vi "Geometry_Util_Test.vi"(8 "error in (no error)":errorcluster) -> (0 "error out":errorcluster, 3 "All Passed":bool)   [LabVIEW 2019]
uses:
  <vilib>/Rock Robotics/WPI/ThirdParty/JAS_Junk/TrajLib/Conv_Deg_Radians.vi
  <vilib>/Rock Robotics/WPI/ThirdParty/JAS_Junk/TrajLib/Rotation2d_CreateAngle.vi
  <vilib>/Rock Robotics/WPI/ThirdParty/JAS_Junk/TrajLib/Rotation2d_GetRadians.vi
  <vilib>/Rock Robotics/WPI/ThirdParty/JAS_Junk/TrajLib/Conv_Radians_Deg.vi
  <vilib>/Rock Robotics/WPI/ThirdParty/MJansen/PathPlanner/PathPlanner.lvlib
  <vilib>/Rock Robotics/WPI/ThirdParty/JAS_Junk/TrajLib/Trajectory_Library.lvlib
panel:
  out "Passed 5":bool
  out "Passed 4":bool
  out "Passed 3":bool
  out "Passed 2":bool
  out "Passed 1":bool
  # "Quadratic LERP"
  # "Double LERP"
  # "Rotational LERP"
  # "Cubic LERP"
  # "Translational LERP"
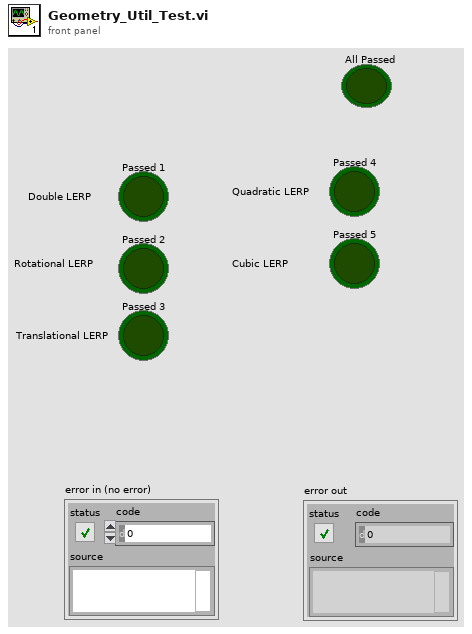
[diagram p1: front panel]
types:
  T1 = typedef "Trajectory_Library.lvlib/TRANSLATION2D.ctl" = cluster{"X":dbl, "Y":dbl}
  T2 = typedef "Trajectory_Library.lvlib/ROTATION2D.ctl" = cluster{"VALUE":dbl, "COS":dbl, "SIN":dbl}
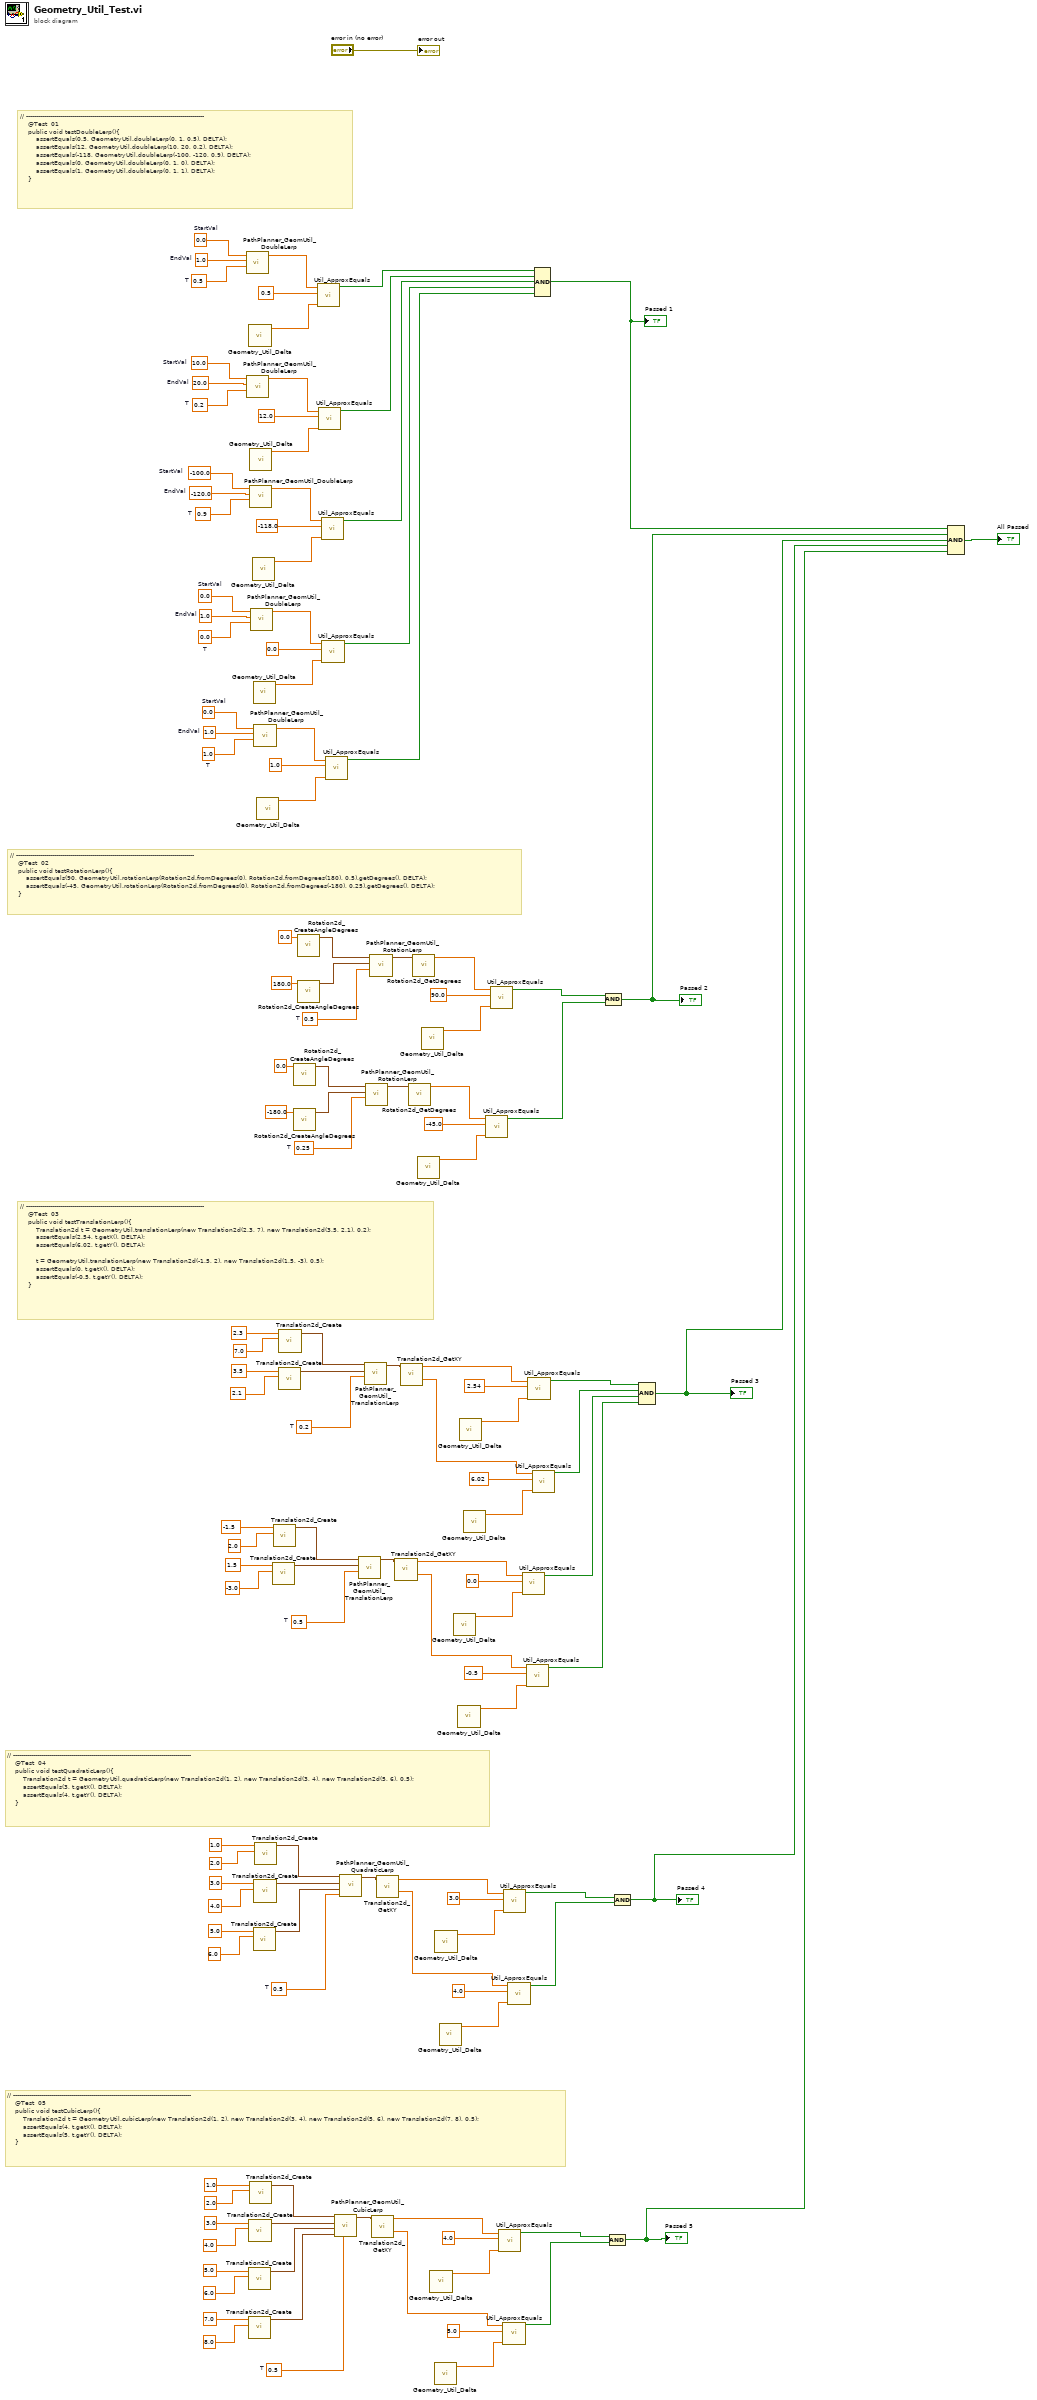
[diagram p0: block diagram]
diagram:
  w21 = 0.5  # T
  w41 = 0.5  # T
  w57 = 0.5  # T
  w74 = 0.2  # T
  w85 = 0.25  # T
  w95 = 0.5  # T
  w103 = 0.0  # StartVal
  w104 = 1.0  # EndVal
  w105 = 1.0  # T
  w109 = 0.0  # StartVal
  w110 = 1.0  # EndVal
  w111 = 0.0  # T
  w115 = -100.0  # StartVal
  w116 = -120.0  # EndVal
  w117 = 0.9  # T
  w121 = 10.0  # StartVal
  w122 = 20.0  # EndVal
  w123 = 0.2  # T
  w128 = 0.0  # StartVal
  w129 = 1.0  # EndVal
  w130 = 0.5  # T
  # "// -----------------------------------------------------------------------------------------\n    @Test  05\n    public void testCubicLerp(){\n        Translation2d t = GeometryUtil.cubicLerp(new Translation2d(1, 2), new Translation2d(3, 4), new Translation2d(5, 6), new Translation2d(7, 8), 0.5);\n        assertEquals(4, t.getX(), DELTA);\n        assertEquals(5, t.getY(), DELTA);\n    }"
  # "// -----------------------------------------------------------------------------------------\n    @Test  04\n    public void testQuadraticLerp(){\n        Translation2d t = GeometryUtil.quadraticLerp(new Translation2d(1, 2), new Translation2d(3, 4), new Translation2d(5, 6), 0.5);\n        assertEquals(3, t.getX(), DELTA);\n        assertEquals(4, t.getY(), DELTA);\n    }"
  # "// -----------------------------------------------------------------------------------------\n    @Test  03\n    public void testTranslationLerp(){\n        Translation2d t = GeometryUtil.translationLerp(new Translation2d(2.3, 7), new Translation2d(3.5, 2.1), 0.2);\n        assertEquals(2.54, t.getX(), DELTA);\n        assertEquals(6.02, t.getY(), DELTA);\n\n        t = GeometryUtil.translationLerp(new Translation2d(-1.5, 2), new Translation2d(1.5, -3), 0.5);\n        assertEquals(0, t.getX(), DELTA);\n        assertEquals(-0.5, t.getY(), DELTA);\n    }"
  # "// -----------------------------------------------------------------------------------------\n    @Test  02\n    public void testRotationLerp(){\n        assertEquals(90, GeometryUtil.rotationLerp(Rotation2d.fromDegrees(0), Rotation2d.fromDegrees(180), 0.5).getDegrees(), DELTA);\n        assertEquals(-45, GeometryUtil.rotationLerp(Rotation2d.fromDegrees(0), Rotation2d.fromDegrees(-180), 0.25).getDegrees(), DELTA);\n    }"
  # "// -----------------------------------------------------------------------------------------\n    @Test  01\n    public void testDoubleLerp(){\n        assertEquals(0.5, GeometryUtil.doubleLerp(0, 1, 0.5), DELTA);\n        assertEquals(12, GeometryUtil.doubleLerp(10, 20, 0.2), DELTA);\n        assertEquals(-118, GeometryUtil.doubleLerp(-100, -120, 0.9), DELTA);\n        assertEquals(0, GeometryUtil.doubleLerp(0, 1, 0), DELTA);\n        assertEquals(1, GeometryUtil.doubleLerp(0, 1, 1), DELTA);\n    }"
  n1 = call <vilib>:"PathPlanner_GeomUtil_DoubleLerp.vi"("T"=w130, "EndVal"=w129, "StartVal"=w128) -> ("Lerp"=w132:dbl)  [unwired: 8 in]
  n2 = call <vilib>:"PathPlanner_GeomUtil_DoubleLerp.vi"("T"=w123, "EndVal"=w122, "StartVal"=w121) -> ("Lerp"=w125:dbl)  [unwired: 8 in]
  n3 = call <vilib>:"Translation2d_Create.vi"("Y"=6.0, "X"=5.0) -> ("TRANSLATION"=w5:T1)  [unwired: 9 in]
  n4 = call <vilib>:"Translation2d_Create.vi"("Y"=8.0, "X"=7.0) -> ("TRANSLATION"=w2:T1)  [unwired: 9 in]
  n5 = call "Geometry_Util_Delta.vi"() -> ("Delta"=w133:dbl)  [unwired: 11 in]
  n6 = call <vilib>:"Translation2d_Create.vi"("Y"=4.0, "X"=3.0) -> ("TRANSLATION"=w14:T1)  [unwired: 9 in]
  n7 = call "Geometry_Util_Delta.vi"() -> ("Delta"=w126:dbl)  [unwired: 11 in]
  n8 = call <vilib>:"PathPlanner_GeomUtil_DoubleLerp.vi"("T"=w117, "EndVal"=w116, "StartVal"=w115) -> ("Lerp"=w119:dbl)  [unwired: 8 in]
  n9 = call <vilib>:"Translation2d_Create.vi"("Y"=2.0, "X"=1.0) -> ("TRANSLATION"=w15:T1)  [unwired: 9 in]
  n10 = call <vilib>:"PathPlanner_GeomUtil_DoubleLerp.vi"("T"=w111, "EndVal"=w110, "StartVal"=w109) -> ("Lerp"=w113:dbl)  [unwired: 8 in]
  n11 = call "Geometry_Util_Delta.vi"() -> ("Delta"=w120:dbl)  [unwired: 11 in]
  n12 = call "Geometry_Util_Delta.vi"() -> ("Delta"=w114:dbl)  [unwired: 11 in]
  n13 = call <vilib>:"Translation2d_Create.vi"("Y"=6.0, "X"=5.0) -> ("TRANSLATION"=w25:T1)  [unwired: 9 in]
  n14 = call <vilib>:"PathPlanner_GeomUtil_DoubleLerp.vi"("T"=w105, "EndVal"=w104, "StartVal"=w103) -> ("Lerp"=w107:dbl)  [unwired: 8 in]
  n15 = call <vilib>:"Translation2d_Create.vi"("Y"=4.0, "X"=3.0) -> ("TRANSLATION"=w34:T1)  [unwired: 9 in]
  n16 = call <vilib>:"Translation2d_Create.vi"("Y"=2.0, "X"=1.0) -> ("TRANSLATION"=w35:T1)  [unwired: 9 in]
  n17 = call "Geometry_Util_Delta.vi"() -> ("Delta"=w108:dbl)  [unwired: 11 in]
  n18 = call <vilib>:"Translation2d_Create.vi"("Y"=-3.0, "X"=1.5) -> ("TRANSLATION"=w50:T1)  [unwired: 9 in]
  n19 = call <vilib>:"Translation2d_Create.vi"("Y"=2.0, "X"=-1.5) -> ("TRANSLATION"=w51:T1)  [unwired: 9 in]
  n20 = call <vilib>:"Translation2d_Create.vi"("Y"=2.1, "X"=3.5) -> ("TRANSLATION"=w67:T1)  [unwired: 9 in]
  n21 = call <vilib>:"Translation2d_Create.vi"("Y"=7.0, "X"=2.3) -> ("TRANSLATION"=w68:T1)  [unwired: 9 in]
  n22 = call <vilib>:"Rotation2d_CreateAngleDegrees.vi"("Angle_Degrees"=0.0) -> ("ROTATION"=w84:T2)  [unwired: 10 in]
  n23 = call <vilib>:"Rotation2d_CreateAngleDegrees.vi"("Angle_Degrees"=-180.0) -> ("ROTATION"=w83:T2)  [unwired: 10 in]
  n24 = call <vilib>:"Rotation2d_CreateAngleDegrees.vi"("Angle_Degrees"=0.0) -> ("ROTATION"=w94:T2)  [unwired: 10 in]
  n25 = call <vilib>:"Rotation2d_CreateAngleDegrees.vi"("Angle_Degrees"=180.0) -> ("ROTATION"=w93:T2)  [unwired: 10 in]
  n26 = call <vilib>:"Util_ApproxEquals.vi"("Tolerance"=w133, "Value 2"=0.5, "Value 1"=w132) -> ("ApproxEquals"=w127:bool)  [unwired: 8 in]
  n27 = call <vilib>:"Util_ApproxEquals.vi"("Tolerance"=w126, "Value 2"=12.0, "Value 1"=w125) -> ("ApproxEquals"=w102:bool)  [unwired: 8 in]
  n28 = call <vilib>:"Util_ApproxEquals.vi"("Tolerance"=w120, "Value 2"=-118.0, "Value 1"=w119) -> ("ApproxEquals"=w101:bool)  [unwired: 8 in]
  n29 = call <vilib>:"Util_ApproxEquals.vi"("Tolerance"=w114, "Value 2"=0.0, "Value 1"=w113) -> ("ApproxEquals"=w100:bool)  [unwired: 8 in]
  n30 = call <vilib>:"Util_ApproxEquals.vi"("Tolerance"=w108, "Value 2"=1.0, "Value 1"=w107) -> ("ApproxEquals"=w99:bool)  [unwired: 8 in]
  n31 = call <vilib>:"PathPlanner_GeomUtil_CubicLerp.vi"("T"=w21, "D"=w2, "C"=w5, "B"=w14, "A"=w15) -> ("Lerp"=w20:T1)  [unwired: 6 in]
  n32 = call <vilib>:"PathPlanner_GeomUtil_QuadraticLerp.vi"("T"=w41, "C"=w25, "B"=w34, "A"=w35) -> ("Lerp"=w40:T1)  [unwired: 7 in]
  n33 = call <vilib>:"PathPlanner_GeomUtil_TranslationLerp.vi"("T"=w57, "EndVal"=w50, "StartVal"=w51) -> ("Lerp"=w56:T1)  [unwired: 8 in]
  n34 = call <vilib>:"PathPlanner_GeomUtil_TranslationLerp.vi"("T"=w74, "EndVal"=w67, "StartVal"=w68) -> ("Lerp"=w73:T1)  [unwired: 8 in]
  n35 = call <vilib>:"PathPlanner_GeomUtil_RotationLerp.vi"("T"=w85, "EndVal"=w83, "StartVal"=w84) -> ("Lerp"=w80:T2)  [unwired: 8 in]
  n36 = call <vilib>:"PathPlanner_GeomUtil_RotationLerp.vi"("T"=w95, "EndVal"=w93, "StartVal"=w94) -> ("Lerp"=w90:T2)  [unwired: 8 in]
  n37 = call <vilib>:"Translation2d_GetXY.vi"("In Translation"=w20) -> ("Y"=w16:dbl, "X"=w19:dbl)  [unwired: 9 in]
  n38 = call <vilib>:"Translation2d_GetXY.vi"("In Translation"=w40) -> ("Y"=w36:dbl, "X"=w39:dbl)  [unwired: 9 in]
  n39 = call <vilib>:"Translation2d_GetXY.vi"("In Translation"=w56) -> ("Y"=w52:dbl, "X"=w55:dbl)  [unwired: 9 in]
  n40 = call <vilib>:"Translation2d_GetXY.vi"("In Translation"=w73) -> ("Y"=w69:dbl, "X"=w72:dbl)  [unwired: 9 in]
  n41 = call <vilib>:"Rotation2d_GetDegrees.vi"("in ROTATION"=w80) -> ("AngleDegrees"=w79:dbl)  [unwired: 10 in]
  n42 = call <vilib>:"Rotation2d_GetDegrees.vi"("in ROTATION"=w90) -> ("AngleDegrees"=w89:dbl)  [unwired: 10 in]
  n43 = call "Geometry_Util_Delta.vi"() -> ("Delta"=w87:dbl)  [unwired: 11 in]
  n44 = call "Geometry_Util_Delta.vi"() -> ("Delta"=w97:dbl)  [unwired: 11 in]
  n45 = call "Geometry_Util_Delta.vi"() -> ("Delta"=w23:dbl)  [unwired: 11 in]
  n46 = call "Geometry_Util_Delta.vi"() -> ("Delta"=w18:dbl)  [unwired: 11 in]
  n47 = call "Geometry_Util_Delta.vi"() -> ("Delta"=w43:dbl)  [unwired: 11 in]
  n48 = call "Geometry_Util_Delta.vi"() -> ("Delta"=w38:dbl)  [unwired: 11 in]
  n49 = call "Geometry_Util_Delta.vi"() -> ("Delta"=w59:dbl)  [unwired: 11 in]
  n50 = call "Geometry_Util_Delta.vi"() -> ("Delta"=w54:dbl)  [unwired: 11 in]
  n51 = call "Geometry_Util_Delta.vi"() -> ("Delta"=w76:dbl)  [unwired: 11 in]
  n52 = call "Geometry_Util_Delta.vi"() -> ("Delta"=w71:dbl)  [unwired: 11 in]
  n53 = call <vilib>:"Util_ApproxEquals.vi"("Tolerance"=w87, "Value 2"=-45.0, "Value 1"=w79) -> ("ApproxEquals"=w78:bool)  [unwired: 8 in]
  n54 = call <vilib>:"Util_ApproxEquals.vi"("Tolerance"=w97, "Value 2"=90.0, "Value 1"=w89) -> ("ApproxEquals"=w88:bool)  [unwired: 8 in]
  n55 = call <vilib>:"Util_ApproxEquals.vi"("Tolerance"=w23, "Value 2"=4.0, "Value 1"=w19) -> ("ApproxEquals"=w9:bool)  [unwired: 8 in]
  n56 = call <vilib>:"Util_ApproxEquals.vi"("Tolerance"=w18, "Value 2"=5.0, "Value 1"=w16) -> ("ApproxEquals"=w8:bool)  [unwired: 8 in]
  n57 = call <vilib>:"Util_ApproxEquals.vi"("Tolerance"=w43, "Value 2"=3.0, "Value 1"=w39) -> ("ApproxEquals"=w29:bool)  [unwired: 8 in]
  n58 = call <vilib>:"Util_ApproxEquals.vi"("Tolerance"=w38, "Value 2"=4.0, "Value 1"=w36) -> ("ApproxEquals"=w28:bool)  [unwired: 8 in]
  n59 = call <vilib>:"Util_ApproxEquals.vi"("Tolerance"=w59, "Value 2"=0.0, "Value 1"=w55) -> ("ApproxEquals"=w45:bool)  [unwired: 8 in]
  n60 = call <vilib>:"Util_ApproxEquals.vi"("Tolerance"=w54, "Value 2"=-0.5, "Value 1"=w52) -> ("ApproxEquals"=w44:bool)  [unwired: 8 in]
  n61 = call <vilib>:"Util_ApproxEquals.vi"("Tolerance"=w76, "Value 2"=2.54, "Value 1"=w72) -> ("ApproxEquals"=w62:bool)  [unwired: 8 in]
  n62 = call <vilib>:"Util_ApproxEquals.vi"("Tolerance"=w71, "Value 2"=6.02, "Value 1"=w69) -> ("ApproxEquals"=w61:bool)  [unwired: 8 in]
  n63 = Compound Arithmetic op=AND(w127, w102, w101, w100, w99) -> (w98:bool)
  "Passed 1" <- w98
  n64 = Compound Arithmetic op=AND(w88, w78) -> (w77:bool)
  "Passed 2" <- w77
  n65 = Compound Arithmetic op=AND(w9, w8) -> (w1:bool)
  "Passed 5" <- w1
  n66 = Compound Arithmetic op=AND(w29, w28) -> (w24:bool)
  "Passed 4" <- w24
  n67 = Compound Arithmetic op=AND(w62, w61, w45, w44) -> (w60:bool)
  "Passed 3" <- w60
  n68 = Compound Arithmetic op=AND(w98, w77, w60, w24, w1) -> (→"All Passed":bool)
  "error out" <- "error in (no error)"
